vi "MeasureQueueCreate.vi"(2 "error in (no error)":errorcluster) -> (0 "MeasureError":errorcluster, 1 "MeasureQueue":refnum<queue>)   [LabVIEW 2017]
uses:
  MeasureQueue.ctl
  MeasureMessage.ctl
panel:
  in  "MeasureQueue":T1
  in  "Queue name":string
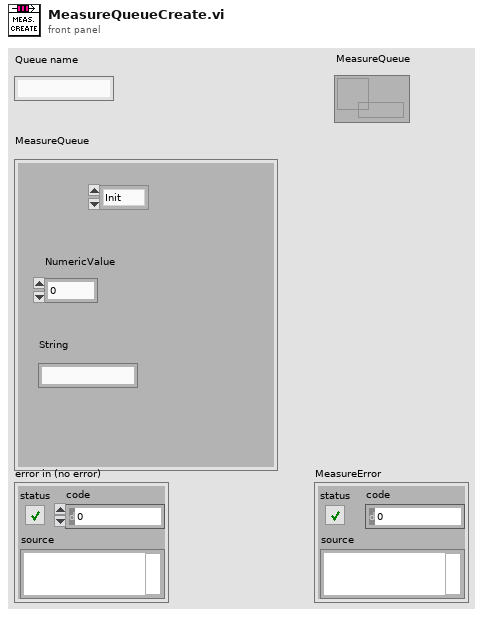
[diagram p1: front panel]
types:
  T1 = typedef "MeasureQueue.ctl" = cluster{"NumericValue":dbl, "String":string, "MeasureMessage":T2}
  T2 = typedef "MeasureMessage.ctl" = enum16{"Init", "Measure", "Error", "Halt", "StartChannel", "StopChannel"}
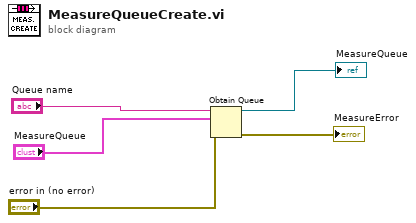
[diagram p0: block diagram]
diagram:
  n1 = Obtain Queue(name (unnamed)="Queue name", element data type="MeasureQueue", error in (no error)="error in (no error)") -> (queue out=→"MeasureQueue":refnum<queue>, error out=→"MeasureError":errorcluster)  [unwired: 2 in, 1 out]
